vi "Update State Connections.vi"(8 "error in (no error)":errorcluster, 9 "connection list":T1[](array[typedef]), 10 "State":string, 11 "Channel Ref in":T2 format="%.0x") -> (0 "error out":errorcluster, 3 "Channel Ref out":T2=18446744073709551615 format="%.0x")   [LabVIEW 2017, in "Switch Scripting.lvlib"]
uses:
  Switch Scripting.lvlib
  <vilib>/NI Veristand/Custom Device API/Custom Device Item Ref.ctl
  Shared/Connection.ctl
  <vilib>/NI VeriStand/Custom Device API/Custom Device API.lvlib
  Shared/Routing and Faulting Shared.lvlib
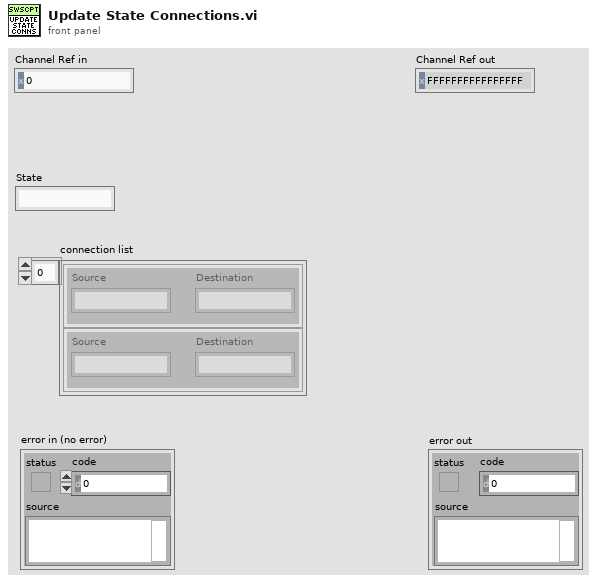
[diagram p1: front panel]
types:
  T1 = typedef "Routing and Faulting Shared.lvlib/Connection.ctl" = cluster{"Source":string, "Destination":string}
  T2 = typedef "Custom Device API.lvlib/Custom Device Item Ref.ctl" = u64
  T3 = typedef "Routing and Faulting Shared.lvlib/Routing State.ctl" = cluster{"Name":string, "Description":string, "Value":i32, "Connection List":T1[]}
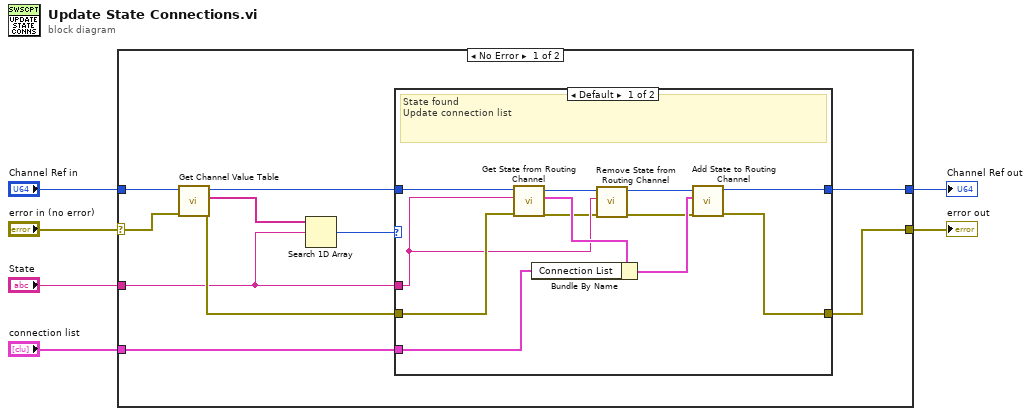
[diagram p0: block diagram]
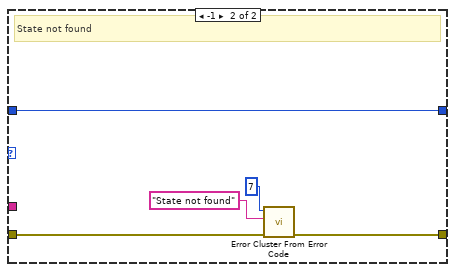
[diagram p2: hidden frame]
diagram:
  n1 = case shown="No Error" "error in (no error)" {
    selector: "error in (no error)" -> [w15 w35]
    tunnel: [w11 w35] -> w1
    tunnel: "Channel Ref in" -> [w16 w34]
    tunnel: [w12 w34] -> w2
    tunnel: "State" -> [w9 _]
    tunnel: "connection list" -> [w7 _]
    frame No Error {
      n2 = call "Get Channel Value Table.vi"("error in (no error)"=w15, "Channel Ref in"=w16) -> ("error out"=w13:errorcluster, "States"=w10:string[], "Channel Ref out"=w14:T2)  [unwired: 6 in, 1 out]
      n3 = Search 1D Array(1D array=w10, element=w9) -> (index of element=w8:i32)  [unwired: 1 in]
      n4 = case shown="Default" w8 {
        tunnel: w14 -> [w28 w30]
        tunnel: w13 -> [w27 w32]
        tunnel: [w18 w30] -> w12
        tunnel: [w17 w31] -> w11
        tunnel: w9 -> [w23 _]
        tunnel: w7 -> [w24 _]
        frame Default {
          # "State found\nUpdate connection list"
          n5 = call "Get State from Routing Channel.vi"("error in (no error)"=w27, "State"=w23, "Channel Ref in"=w28) -> ("error out"=w20:errorcluster, "Routing State"=w26:T3, "Channel Ref out"=w22:T2)  [unwired: 6 in]
          n6 = Bundle By Name(cluster=w26, "Connection List"=w24) -> (w25:T3)
          n7 = call "Remove State from Routing Channel.vi"("error in (no error)"=w20, "State"=w23, "Channel Ref in"=w22) -> ("error out"=w19:errorcluster, "Channel Ref out"=w21:T2)  [unwired: 7 in]
          n8 = call "Add State to Routing Channel.vi"("error in (no error)"=w19, "Routing State"=w25, "Channel Ref in"=w21) -> ("error out"=w17:errorcluster, "Channel Ref out"=w18:T2)  [unwired: 7 in]
        }
        frame -1 {
          # "State not found"
          n9 = call <vilib>:"Error Cluster From Error Code.vi"("error in (no error)"=w32, "error message (\"\")"="State not found" ("error message (\"\")"), "error code (0)"=7) -> ("error out"=w31:errorcluster)  [unwired: 6 in]
        }
      }
    }
    frame Error {
    }
  }
  "Channel Ref out" <- w2
  "error out" <- w1
